vi "tt20_relable_chart_legends.vi"(8 "error in (no error)":errorcluster, 10 "panel in":refnum<class "panel.lvclass">, 11 "tt20 in":refnum<class "tt20.lvclass">) -> (0 "error out":errorcluster, 2 "panel out":refnum<class "panel.lvclass">, 3 "tt20 out":refnum<class "tt20.lvclass">)   [LabVIEW 2015, in "tt20.lvclass"]
uses:
  tt20.lvclass
  UI/panel_class/panel.lvclass
  UI/panel_class/panel.lvclass/panel.ctl
  tt20.lvclass/tt20.ctl
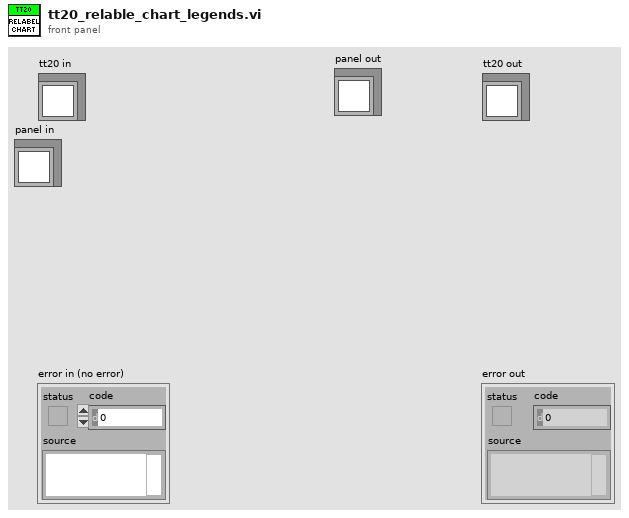
[diagram p1: front panel]
types:
  T1 = typedef "ui_plot_references.ctl" = cluster{"plots":refnum<vi>, "chart":refnum<vi>, "graph":refnum<vi>, "map":refnum<vi>, "XY Graph":refnum<vi>}
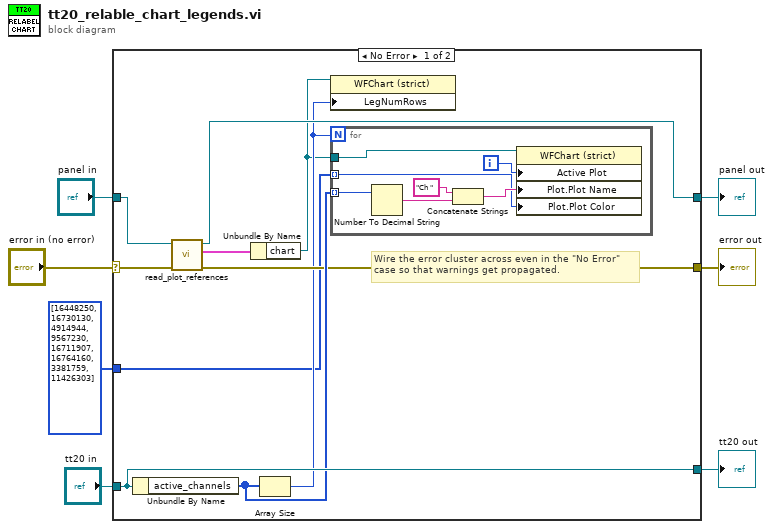
[diagram p0: block diagram]
diagram:
  n1 = case shown="No Error" "error in (no error)" {
    selector: "error in (no error)" -> [w13 w27]
    tunnel: [w12 w27] -> w6
    tunnel: [w15 w26] -> w4
    tunnel: "tt20 in" -> [w15 w26]
    tunnel: "panel in" -> [w17 w25]
    tunnel: [w11 w25] -> w2
    tunnel: u32[] [16448250, 16730130, 4914944, 9567230, 16711907, 16764160, 3381759, 11426303] -> [w8 _]
    frame No Error {
      # "Wire the error cluster across even in the \"No Error\"\ncase so that warnings get propagated."
      n2 = Unbundle By Name(w15) -> ("active_channels"=w14:u32[])
      n3 = call "read_plot_references.vi"("error in (no error)"=w13, "panel in"=w17) -> ("error out"=w12:errorcluster, "plot_references"=w16:T1, "panel out"=w11:refnum<class "panel.lvclass">)  [unwired: 7 in]
      n4 = Unbundle By Name(w16) -> ("chart"=w9:refnum<vi>)
      n5 = Array Size(array=w14) -> (size(s)=w10:i32)
      n6 = property class="WFChart (strict)"(reference=w9, "LegNumRows"=w10) -> ()  [unwired: 1 in, 2 out]
      n7 = for {
        N: w10 -> [_]
        tunnel: w9 -> [w24]
        tunnel: w14 -> [w19] mode=indexing
        tunnel: w8 -> [w18] mode=indexing
        i -> [w23]
        n8 = Number To Decimal String(number=w19) -> (decimal integer string=w21:string)  [unwired: 1 in]
        n9 = Concatenate Strings("Ch ", w21) -> (w20:string)
        n10 = property class="WFChart (strict)"(reference=w24, "Active Plot"=w23, "Plot.Plot Name"=w20, "Plot.Plot Color"=w18) -> ()  [unwired: 1 in, 2 out]
      }
    }
    frame Error {
    }
  }
  "error out" <- w6
  "tt20 out" <- w4
  "panel out" <- w2
